vi "ep02_subvi.vi"() -> ()   [LabVIEW 2019]
panel:
  out "Information":string
  out "Port Status":bool
  in  "Baud Rate Input":T1(ring)=enum."115200" caption="Baud Rate"
  in  "Port Id Input":T2(ring) caption="Port Name"
  in  "stop":bool
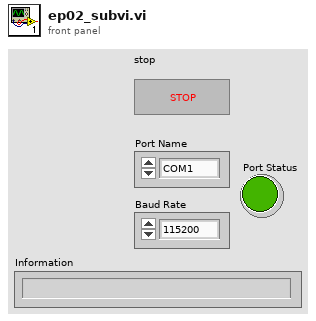
[diagram p1: front panel]
types:
  T1 = enum32{"300", "600", "1200", "2400", "4800", "9600", "14400", "19200", "28800", "38400", "56000", "57600", "115200", "128000", "256000"}
  T2 = enum8{"COM1", "COM2", "COM3", "COM4", "COM5", "COM6", "COM7", "COM8", "COM9", "COM10", "COM11", "COM12", "COM13", "COM14", "COM15", "COM16", "COM17", "COM18", "COM19", "COM20", "COM21", "COM22", "COM23", "COM24", "COM25", "COM26", "COM27", "COM28", "COM29", "COM30", "COM31", "COM32", "COM33", "COM34", "COM35", "COM36", "COM37", "COM38", "COM39", "COM40", "COM41", "COM42", "COM43", "COM44", "COM45", "COM46", "COM47", "COM48"}
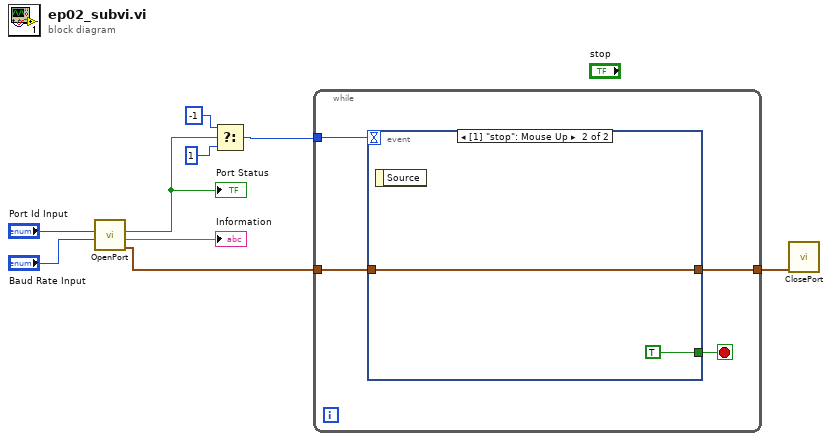
[diagram p0: block diagram]
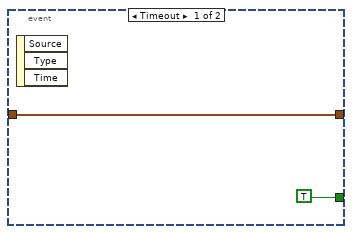
[diagram p2: hidden frame]
diagram:
  n1 = call "OpenPort.vi"("Baud Rate Input"="Baud Rate Input", "Port Id Input"="Port Id Input") -> ("Uart Output"=w6:cluster{u64}, "Information"=→"Information":string, "Port Status"=w1:bool)  [unwired: 6 in, 1 out]
  "Port Status" <- w1
  n2 = Select(t=-1, s=w1, f=1) -> (s? t:f=w3:i32)
  n3 = while {
    tunnel: w6 -> [w10]
    tunnel: [w12] -> w5
    tunnel: w3 -> [w11]
    stop <- w13 stop-if-true
    n4 = event shown="[1] \"stop\": Mouse Up" {
      selector: _ -> [_ _]
      dyn-events: _ -> [_ _]
      timeout: w11 -> [_ _]
      tunnel: [TRUE TRUE] -> w13
      tunnel: w10 -> [w14 w16]
      tunnel: [w14 w16] -> w12
      event Timeout {
        n5 = event-data() -> ()  [unwired: 1 in, 3 out]
      }
      event "stop": Mouse Up {
        n6 = event-data() -> ()  [unwired: 1 in, 1 out]
      }
    }
  }
  n7 = call "ClosePort.vi"("Uart Input"=w5) -> ()  [unwired: 9 in, 2 out]
